vi "measure_signal.vi"(8 "error in":errorcluster, 10 "Measurement settings":T1={"Start Wavelength (nm)"=300.0, "End Wavelength (nm)"=900.0, "Increment (nm)"=5.0, "White Bias"="Off", "Averages per wavlength"=1.0, "Time Constant"=8, "Low Pass Filter Slope "=1, "Gain (V/A)"=50.0, "Ratio mode"="On"} {"Gain (V/A)" format="%#.2f"; "Low Pass Filter Slope" items=["6 dB/oct", "12 dB/oct", "18 db/oct", "24 dB/oct"]; "Time Constant" items=["10 us", "30 us", "100 us", "300 us", "1 ms", "3 ms", "10 ms", "30 ms", "100 ms", "300 ms", "1 s", "3 s", "10 s", "30 s", "100 s", "300 s", "1 ks", "3 ks", "10 ks", "30 ks"]; "Averages per wavlength" format="%#.2f"; "End Wavelength (nm)" min=350.0 max=1100.0 format="%#.2f"; "Start Wavelength (nm)" min=350.0 max=1100.0 format="%#.2f"}, 11 "VISA resource name in":refnum<visa-resource-name>="GPIB0::8::INSTR") -> (0 "error out":errorcluster, 1 "Averaged theta":dbl, 2 "Averaged scaled signal":dbl, 3 "VISA resource name out":refnum<visa-resource-name>)   [LabVIEW 2018]
uses:
  typedefs/measurement_settings.ctl
  <instrlib>/Stanford Research 830/Public/Data/Read (All Parameters).vi
  <instrlib>/Stanford Research 830/Stanford Research 830.lvlib
panel:
  out "Raw signal":dbl
  out "Intensity-graph":T2(graph)
  out "Signal":dbl
  # "Wavelength average intensity"
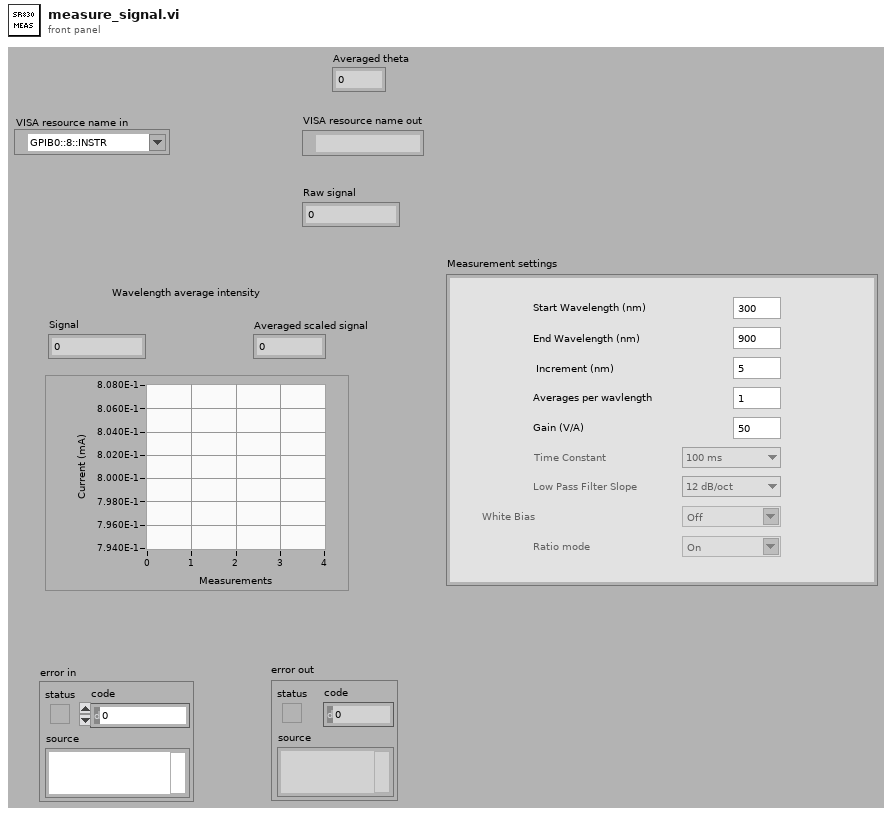
[diagram p1: front panel]
types:
  T1 = typedef "measurement_settings.ctl" = cluster{"Start Wavelength (nm)":dbl, "End Wavelength (nm)":dbl, "Increment (nm)":dbl, "White Bias":string, "Averages per wavlength":dbl, "Time Constant":u16, "Low Pass Filter Slope ":u16, "Gain (V/A)":dbl, "Ratio mode":string}
  T2 = cluster{"meas_index 2":i32[], "Intensity 3":dbl[]}
  T3 = cluster{"X-Value":dbl, "Y-Value":dbl, "R-Value":dbl, "Theta-Value":dbl, "Aux In 1 Value":dbl, "Aux In 2 Value":dbl, "Aux In 3 Value":dbl, "Aux In 4 Value":dbl, "Reference Frequency":dbl, "Channel 1 Display":dbl, "Channel 2 Display":dbl}
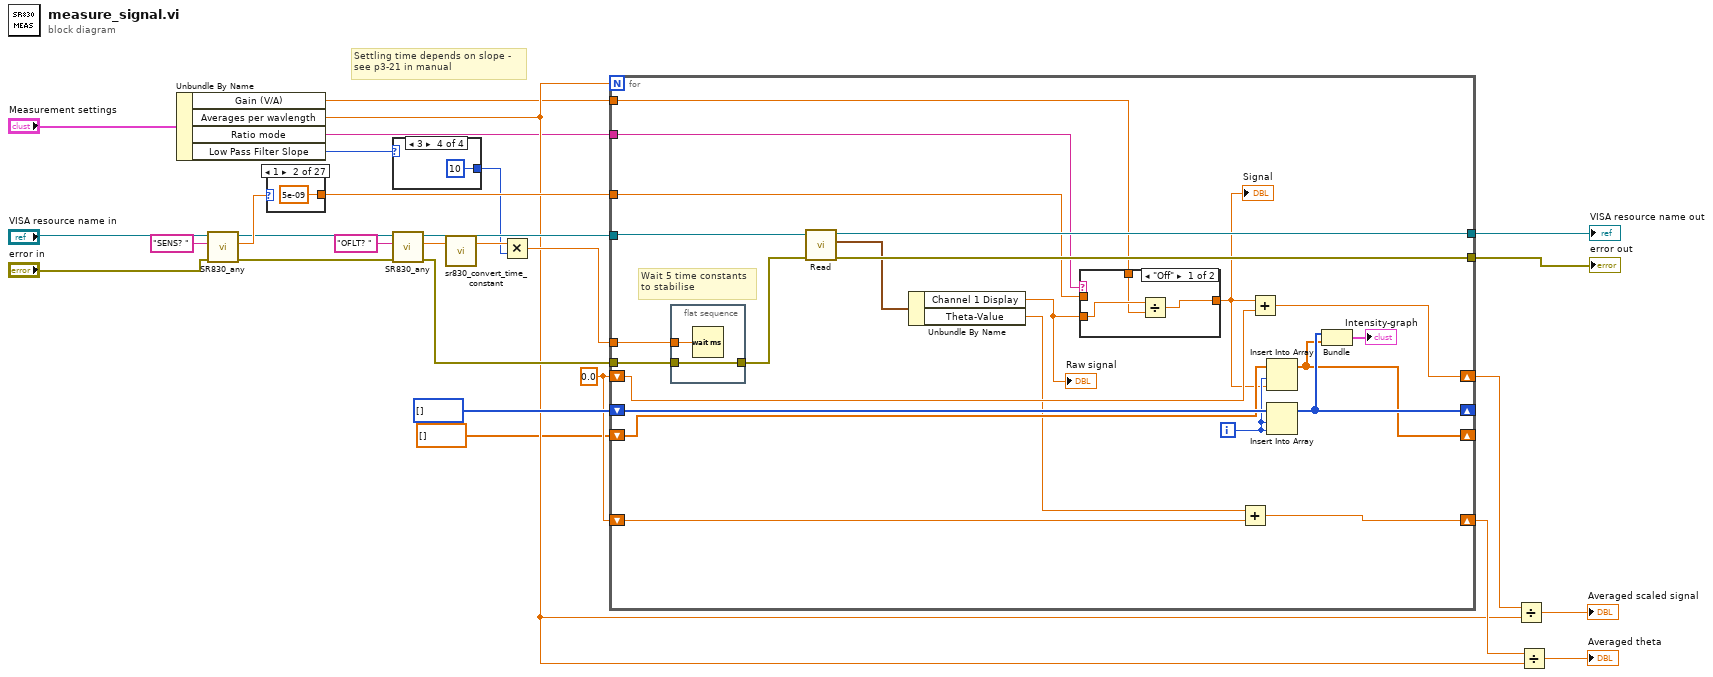
[diagram p0: block diagram]
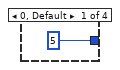
[diagram p2: hidden frame]
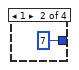
[diagram p3: hidden frame]
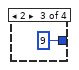
[diagram p4: hidden frame]
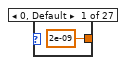
[diagram p5: hidden frame]
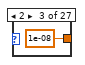
[diagram p6: hidden frame]
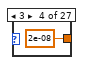
[diagram p7: hidden frame]
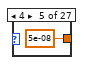
[diagram p8: hidden frame]
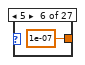
[diagram p9: hidden frame]
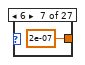
[diagram p10: hidden frame]
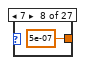
[diagram p11: hidden frame]
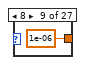
[diagram p12: hidden frame]
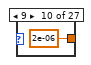
[diagram p13: hidden frame]
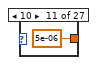
[diagram p14: hidden frame]
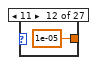
[diagram p15: hidden frame]
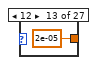
[diagram p16: hidden frame]
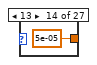
[diagram p17: hidden frame]
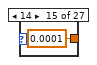
[diagram p18: hidden frame]
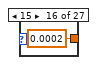
[diagram p19: hidden frame]
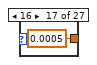
[diagram p20: hidden frame]
diagram:
  w9 = 0.0
  # "Settling time depends on slope -\nsee p3-21 in manual"
  n1 = Unbundle By Name("Measurement settings") -> ("Gain (V/A)"=w3:dbl, "Averages per wavlength"=w7:dbl, "Ratio mode"=w4:string, "Low Pass Filter Slope"=w2:u16)
  n2 = call "SR830_any.vi"("error in (no error)"="error in", "initial string"="SENS? ", "VISA resource name"="VISA resource name in") -> ("error out"=w13:errorcluster, "Measurement"=w15:dbl, "VISA resource name out"=w14:refnum<visa-resource-name>)  [unwired: 6 in]
  n3 = case shown="1" w15 {
    tunnel: [2e-09 5e-09 1e-08 2e-08 5e-08 1e-07 2e-07 5e-07 1e-06 2e-06 5e-06 1e-05 2e-05 5e-05 0.0001 0.0002 0.0005 0.001 0.002 0.005 0.01 0.02 0.05 0.1 0.2 0.5 1] -> w10
    frame 0, Default {
    }
    frame 1 {
    }
    frame 2 {
    }
    frame 3 {
    }
    frame 4 {
    }
    frame 5 {
    }
    frame 6 {
    }
    frame 7 {
    }
    frame 8 {
    }
    frame 9 {
    }
    frame 10 {
    }
    frame 11 {
    }
    frame 12 {
    }
    frame 13 {
    }
    frame 14 {
    }
    frame 15 {
    }
    frame 16 {
    }
    frame 17 {
    }
    frame 18 {
    }
    frame 19 {
    }
    frame 20 {
    }
    frame 21 {
    }
    frame 22 {
    }
    frame 23 {
    }
    frame 24 {
    }
    frame 25 {
    }
    frame 26 {
    }
  }
  n4 = case shown="3" w2 {
    tunnel: [5 7 9 10] -> w1
    frame 0, Default {
    }
    frame 1 {
    }
    frame 2 {
    }
    frame 3 {
    }
  }
  n5 = call "SR830_any.vi"("error in (no error)"=w13, "initial string"="OFLT? ", "VISA resource name"=w14) -> ("error out"=w21:errorcluster, "Measurement"=w22:dbl, "VISA resource name out"=w17:refnum<visa-resource-name>)  [unwired: 6 in]
  n6 = call "sr830_convert_time_constant.vi"("Time constant code"=w22) -> ("time constant  in ms"=w25:dbl)  [unwired: 2 in]
  n7 = Multiply(x=w25, y=w1) -> (x*y=w24:dbl)
  n8 = for {
    N: w7 -> [_]
    tunnel: w17 -> [w70]
    tunnel: [w69] -> w27
    tunnel: [w82] -> w26
    shift-right: [w77] -> w20
    shift-left: w9 -> [w74]
    shift-right: [w76] -> _
    shift-left: i32[] [] -> [w81]
    shift-right: [w75] -> _
    shift-left: dbl[] [] -> [w80]
    tunnel: w24 -> [w73]
    tunnel: w21 -> [w72]
    tunnel: w10 -> [w68]
    shift-right: [w62] -> w8
    shift-left: w9 -> [w63]
    tunnel: w4 -> [w61]
    tunnel: w3 -> [w60]
    i -> [w79]
    # "Wait 5 time constants\nto stabilise"
    n9 = flat-sequence {
      tunnel: w73 -> [w92]
      tunnel: w72 -> [w91]
      tunnel: [w91] -> w71
      frame #0 {
        n10 = Wait (ms)(milliseconds to wait=w92) -> ()  [unwired: 1 out]
      }
    }
    n11 = call-poly <instrlib>:"Read.vi"("error in (no error)"=w71, "VISA resource name"=w70) -> ("error out"=w82:errorcluster, "Parameter Values"=w66:T3, "VISA resource name out"=w69:refnum<visa-resource-name>)  [unwired: 7 in]
    n12 = Unbundle By Name(w66) -> ("Channel 1 Display"=w65:dbl, "Theta-Value"=w64:dbl)
    "Raw signal" <- w65
    n13 = case shown="\"Off\"" w61 {
      tunnel: w68 -> [_ w90]
      tunnel: [w83 w89] -> w67
      tunnel: w65 -> [w85 w86]
      tunnel: w60 -> [w84 _]
      frame "Off" {
        n14 = Divide(x=w85, y=w84) -> (x/y=w83:dbl)
      }
      frame "On", Default {
        n15 = Divide(x=w86, y=1000.0) -> (x/y=w88:dbl)
        n16 = Compound Arithmetic op=MULTIPLY(w90, w88) -> (w89:dbl)
      }
    }
    "Signal" <- w67
    n17 = Add(x=w64, y=w63) -> (x+y=w62:dbl)
    n18 = Add(x=w67, y=w74) -> (x+y=w77:dbl)
    n19 = Insert Into Array(array=w80, index=w79, new element=w67) -> (w75:dbl[])
    n20 = Insert Into Array(array=w81, index=w79, new element=w79) -> (w76:i32[])
    n21 = Bundle(w76, w75) -> (→"Intensity-graph":cluster{i32[], dbl[]})  [unwired: 1 in]
  }
  "VISA resource name out" <- w27
  "error out" <- w26
  n22 = Divide(x=w20, y=w7) -> (x/y=→"Averaged scaled signal":dbl)
  n23 = Divide(x=w8, y=w7) -> (x/y=→"Averaged theta":dbl)
